vi "p-source-coils_Wrapper.vi"(0 "String Array":string[](array[string])=["C:\\CuspControl\\GPIB and Network\\p-coils.txt", "6723"], 1 "Boolean input Array":dbl[](array[numeric])=[0.0]) -> ()   [LabVIEW 2018]
uses:
  <vilib>/Analysis/1siggen.llb/Ramp Pattern by Samples.vi
  <vilib>/DAQmx/write.llb/DAQmx Write (Analog 2D DBL NChan NSamp).vi
  <vilib>/DAQmx/create/channels.llb/DAQmx Create Channel (AO-Voltage-Basic).vi
  <vilib>/DAQmx/configure/timing.llb/DAQmx Timing (Sample Clock).vi
  <vilib>/DAQmx/miscellaneous.llb/DAQmx Fill In Error Info.vi
  <vilib>/Analysis/NI_AALBase.lvlib
panel:
  out "Elapsed time (ms)":u32=106
  in  "rate (S/s)":dbl=1000.0 format="%0.2f"
  in  "samples":i32=100
  out "Enable TL?":bool
  out "Start Values":dbl[](array[numeric])=[10.0, 2.8, 6.3, 5.0, 4.0, 5.6]
  out "End Values":dbl[](array[numeric])
  out "Set Values":dbl[](array[numeric])=[10.0, 2.8, 6.3, 5.0, 4.0, 5.6]
  out "Device names":string[](array[string])=["Dev1/ao0", "Dev1/ao2 ", "Dev1/ao3 "]
  out "# Coils":i32=3
  out "array":dbl[][](array[numeric])=[[10.0, 2.8, 6.3, 5.0, 4.0, 5.6], [0.0, 0.0, 0.0, 0.0, 0.0, 0.0], [0.0, 0.0, 0.0, 0.0, 0.0, 0.0], [0.0, 0.0, 0.0, 0.0, 0.0, 0.0], [0.0, 0.0, 0.0, 0.0, 0.0, 0.0], [0.0, 0.0, 0.0, 0.0, 0.0, 0.0], [0.0, 0.0, 0.0, 0.0, 0.0, 0.0], [0.0, 0.0, 0.0, 0.0, 0.0, 0.0]]
  out "subarray":dbl[](array[numeric])=[10.0, 2.8, 6.3, 5.0, 4.0, 5.6]
  in  "subvi?":bool=TRUE
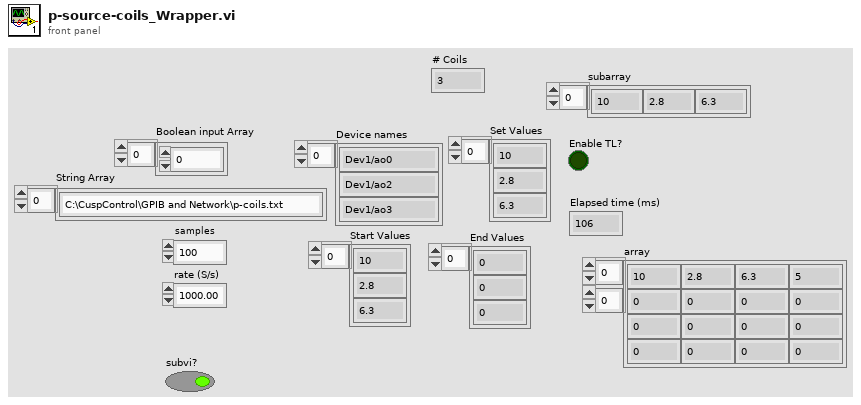
[diagram p1: front panel]
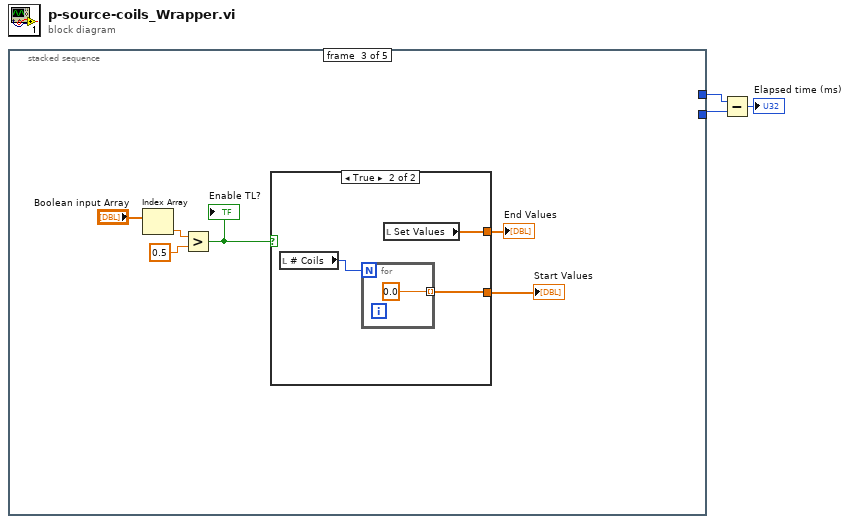
[diagram p0: block diagram]
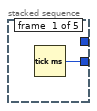
[diagram p2: hidden frame]
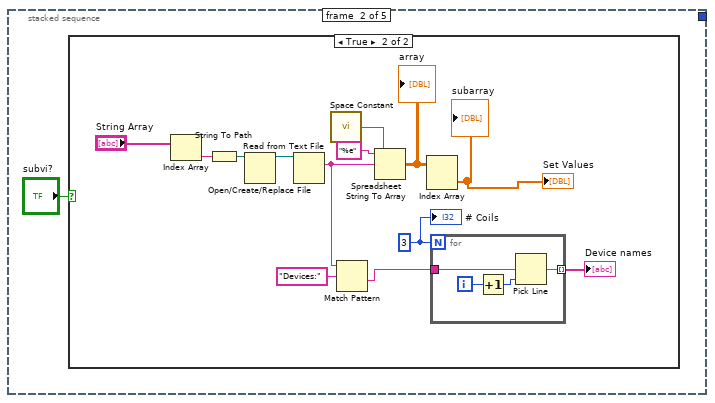
[diagram p3: hidden frame]
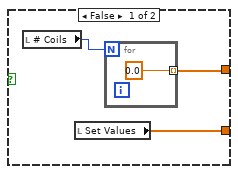
[diagram p5: hidden frame]
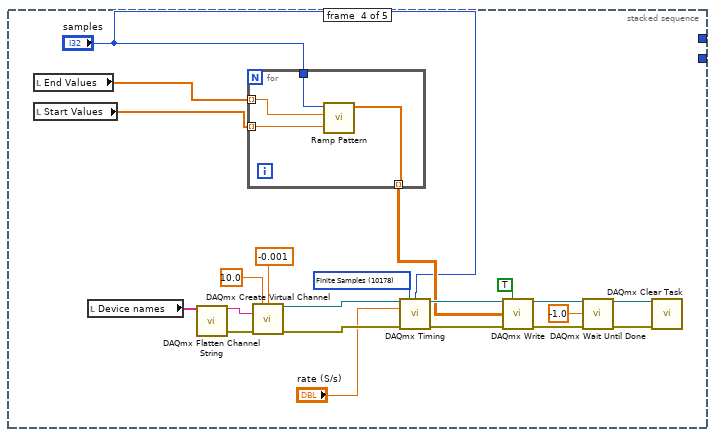
[diagram p6: hidden frame]
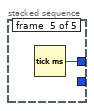
[diagram p7: hidden frame]
diagram:
  n1 = stacked-sequence {
    tunnel: [w4 _ _ _ _] -> w3
    tunnel: [_ _ _ _ w62] -> w2
    frame #0 {
      n2 = Tick Count (ms)() -> (millisecond timer value=w4:u32)
    }
    frame #1 {
      n3 = case shown="True" "subvi?" {
        frame False {
        }
        frame True {
          w7 = 3
          n4 = Index Array(array="String Array") -> (element=w17:string)  [unwired: 1 in]
          n5 = String To Path(string=w17) -> (path=w8:path)
          n6 = Open/Create/Replace File(file path (use dialog)=w8) -> (refnum out=w9:refnum<file>)  [unwired: 5 in, 2 out]
          n7 = Read from Text File(file (use dialog)=w9) -> (text=w13:string)  [unwired: 3 in, 3 out]
          n8 = call <vilib>:"Space Constant.vi"() -> ("String"=w15:string)
          n9 = Match Pattern(string=w13, regular expression="Devices:") -> (after substring=w11:string)  [unwired: 1 in, 3 out]
          n10 = Spreadsheet String To Array(delimiter (Tab)=w15, format string="%e", spreadsheet string=w13) -> (array=w14:dbl[][])  [unwired: 1 in]
          "array" <- w14
          n11 = Index Array(array=w14) -> (element=→"Set Values" →"subarray":dbl[])  [unwired: 2 in]
          n12 = for {
            N: w7 -> [_]
            tunnel: w11 -> [w20]
            tunnel: [w19] -> w10 mode=indexing
            i -> [w22]
            n13 = Increment(x=w22) -> (x+1=w21:i32)
            n14 = Pick Line(multi-line string=w20, line index=w21) -> (output string=w19:string)  [unwired: 1 in]
          }
          "Device names" <- w10
          "# Coils" <- w7
        }
      }
    }
    frame #2 {
      n15 = Index Array(array="Boolean input Array") -> (element=w27:dbl)  [unwired: 1 in]
      n16 = Greater?(x=w27, y=0.5) -> (0:w25:bool)
      "Enable TL?" <- w25
      n17 = case shown="True" w25 {
        tunnel: [w30 w35] -> w23
        tunnel: [w29 w33] -> w24
        frame False {
          n18 = local read "# Coils"() -> (w31:i32)
          n19 = local read "Set Values"() -> (w29:dbl[])
          n20 = for {
            N: w31 -> [_]
            tunnel: [0.0] -> w30 mode=indexing
          }
        }
        frame True {
          n21 = local read "# Coils"() -> (w34:i32)
          n22 = for {
            N: w34 -> [_]
            tunnel: [0.0] -> w33 mode=indexing
          }
          n23 = local read "Set Values"() -> (w35:dbl[])
        }
      }
      "Start Values" <- w24
      "End Values" <- w23
    }
    frame #3 {
      w42 = 10178 items=["Finite Samples"=10178, "Continuous Samples"=10123, "Hardware Timed Single Point"=12522] ("sample mode")
      n24 = local read "End Values"() -> (w40:dbl[])
      n25 = local read "Start Values"() -> (w39:dbl[])
      n26 = local read "Device names"() -> (w37:string[])
      n27 = call <vilib>:"DAQmx Flatten Channel String.vi"("names in"=w37) -> ("names out"=w41:string, "error out"=w48:errorcluster)  [unwired: 13 in]
      n28 = for {
        tunnel: w40 -> [w61] mode=indexing
        tunnel: "samples" -> [w60]
        tunnel: [w59] -> w45 mode=indexing
        tunnel: w39 -> [w58] mode=indexing
        n29 = call-poly <vilib>:"Ramp Pattern.vi"("start"=w58, "end"=w61, "samples"=w60) -> ("Ramp Pattern"=w59:dbl[])  [unwired: 7 in, 1 out]
      }
      n30 = call-poly <vilib>:"DAQmx Create Virtual Channel.vi"("maximum value"=10.0, "minimum value"=-0.001, "physical channels"=w41, "error in"=w48) -> ("task out"=w53:refnum<k21>, "error out"=w54:errorcluster)  [unwired: 10 in]
      n31 = call-poly <vilib>:"DAQmx Timing.vi"("task/channels in"=w53, "sample mode"=w42, "samples per channel"="samples", "rate"="rate (S/s)", "error in"=w54) -> ("task out"=w56:refnum<k21>, "error out"=w55:errorcluster)  [unwired: 9 in]
      n32 = call-poly <vilib>:"DAQmx Write.vi"("task/channels in"=w56, "auto start"=TRUE, "data"=w45, "error in"=w55) -> ("task out"=w52:refnum<k21>, "error out"=w51:errorcluster)  [unwired: 9 in, 1 out]
      n33 = call <vilib>:"DAQmx Wait Until Done.vi"("task/channels in"=w52, "timeout (sec)"=-1.0, "error in"=w51) -> ("task out"=w50:refnum<k21>, "error out"=w49:errorcluster)  [unwired: 11 in]
      n34 = call <vilib>:"DAQmx Clear Task.vi"("task in"=w50, "error in"=w49) -> ()  [unwired: 13 in, 1 out]
    }
    frame #4 {
      n35 = Tick Count (ms)() -> (millisecond timer value=w62:u32)
    }
  }
  n36 = Subtract(x=w2, y=w3) -> (x-y=→"Elapsed time (ms)":u32)
